vi "test_OneSessTwoPinOneInstrTwoSiteReservation_CallNiDigitalGetConnectionsNPinsMConnections_ReturnsThreeConnections.vi"(8 "error in":errorcluster) -> (0 "error out":errorcluster, 2 "result":string, 3 "pass":bool)   [LabVIEW 2020, in "MeasurementServerTests.lvlib"]
uses:
  MeasurementServerTests.lvlib
  Runtime/APIs/Session Management V1/Session Reservation/Connection.ctl
  Runtime/APIs/Session Management V1/Session Reservation/Session Reservation.lvclass
  03fc85e1-696b-4ece-a78b-f41470766ac0.vi
  a536e905-e99b-4ce6-9f7b-add65bd26abc.vi
  f2d0f46c-20cf-4e81-b3a3-5c4fc317eda1.vi
  Runtime/Sessions/niDigital Sessions/Connection with Session.ctl
  Runtime/Sessions/niDigital Sessions/Plug-In SDK niDigital Sessions.lvlib
  Runtime/Sessions/niDigital Sessions/Get Connections - NPin MConn.vi
  9fa65f91-1ac8-4868-844f-6b0c70994850.vi
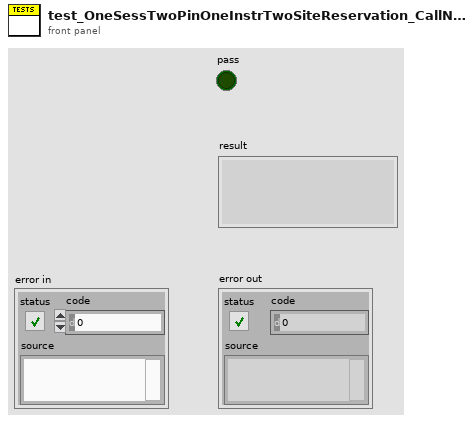
[diagram p1: front panel]
types:
  T1 = typedef "Plug-In SDK niDigital Sessions.lvlib/Connection with Session.ctl" = cluster{"connection":T2, "session":refnum<k15>}
  T2 = typedef "Plug-In SDK Session Management V1 API.lvlib/Session Reservation.lvclass/Connection.ctl" = cluster{"pin or relay name":string, "site":i32, "instrument type id":string, "channel":string}
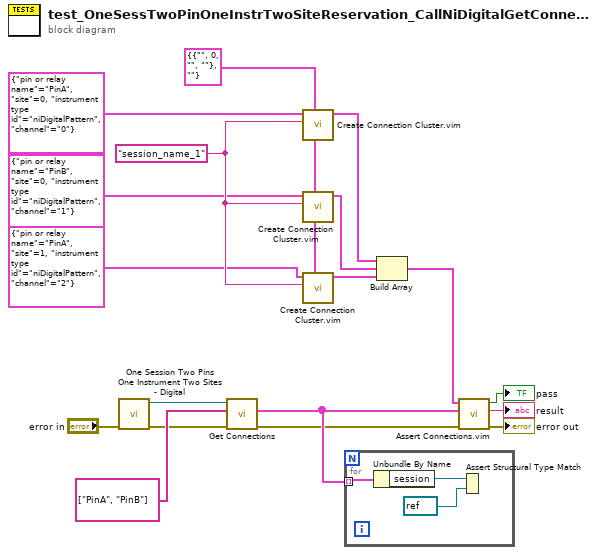
[diagram p0: block diagram]
diagram:
  w8 = T1 {"connection"={"pin or relay name"="", "site"=0, "instrument type id"="", "channel"=""}, "session"=""} ("connection with session")
  w13 = "session_name_1" ("session in")
  n1 = call "One Session Two Pins One Instrument Two Sites - Digital.vi"("error in"="error in") -> ("error out"=w4:errorcluster, "session reservation out"=w3:refnum<class "Session Reservation.lvclass">)  [unwired: 9 in]
  n2 = call-poly "Get Connections.vi"("error in"=w4, "pin or relay names"=string[] ["PinA", "PinB"], "session reservation in"=w3) -> ("error out"=w2:errorcluster, "connections"=w7:T1[])  [unwired: 6 in, 1 out]
  n3 = call "Create Connection Cluster.vim"("connection type"=w8, "session in"=w13, "hardware independent connection in"=T2 {"pin or relay name"="PinA", "site"=0, "instrument type id"="niDigitalPattern", "channel"="0"} ("connection")) -> ("connection out"=w15:T1)  [unwired: 8 in]
  n4 = call "Create Connection Cluster.vim"("connection type"=w8, "session in"=w13, "hardware independent connection in"=T2 {"pin or relay name"="PinB", "site"=0, "instrument type id"="niDigitalPattern", "channel"="1"} ("connection")) -> ("connection out"=w9:T1)  [unwired: 8 in]
  n5 = call "Create Connection Cluster.vim"("connection type"=w8, "session in"=w13, "hardware independent connection in"=T2 {"pin or relay name"="PinA", "site"=1, "instrument type id"="niDigitalPattern", "channel"="2"} ("connection")) -> ("connection out"=w10:T1)  [unwired: 8 in]
  n6 = for {
    tunnel: w7 -> [w19] mode=indexing
    n7 = Unbundle By Name(w19) -> ("session"=w21:refnum<k15>)
    n8 = Assert Structural Type Match(0:refnum<k15> refnum ("session"), 1:w21) -> ()
  }
  n9 = Build Array(w15, w9, w10) -> (w14:T1[])
  n10 = call "Assert Connections.vim"("error in"=w2, "actual connections"=w7, "expected connections"=w14) -> ("error out"=→"error out":errorcluster, "result"=→"result":string, "pass"=→"pass":bool)  [unwired: 6 in]
